vi "Latihan 7 (Shift Register).vi"() -> ()   [LabVIEW 2021]
panel:
  in  "stop":bool
  out "Numeric 2":dbl
  out "Numeric":dbl
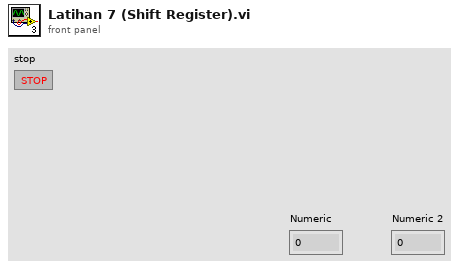
[diagram p1: front panel]
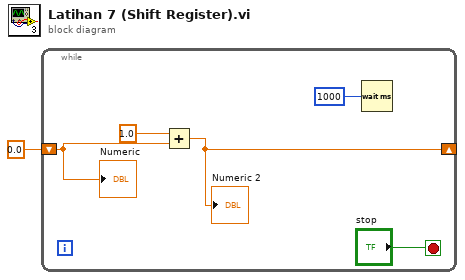
[diagram p0: block diagram]
diagram:
  n1 = while {
    shift-right: [w5] -> _
    shift-left: 0.0 -> [w4]
    stop <- "stop" stop-if-true
    n2 = Add(x=1.0, y=w4) -> (x+y=w5:dbl)
    "Numeric 2" <- w5
    n3 = Wait (ms)(milliseconds to wait=u32 1000) -> ()  [unwired: 1 out]
    "Numeric" <- w4
  }
